vi "Check Default Plugins.vi"(8 "error in (no error)":errorcluster, 11 "Configuration Manager in":refnum<class "Configuration Manager.lvclass">) -> (0 "error out":errorcluster, 3 "Configuration Manager out":refnum<class "Configuration Manager.lvclass">)   [LabVIEW 2020, in "Configuration Manager.lvclass"]
uses:
  Configuration Manager.lvclass
  Configuration Manager.lvclass/Configuration Manager.ctl
  <vilib>/Utility/config.llb/NI_LVConfig.lvlib
  <vilib>/Utility/config.llb/Read Key (Boolean).vi
  <vilib>/Utility/config.llb/Write Key (Boolean).vi
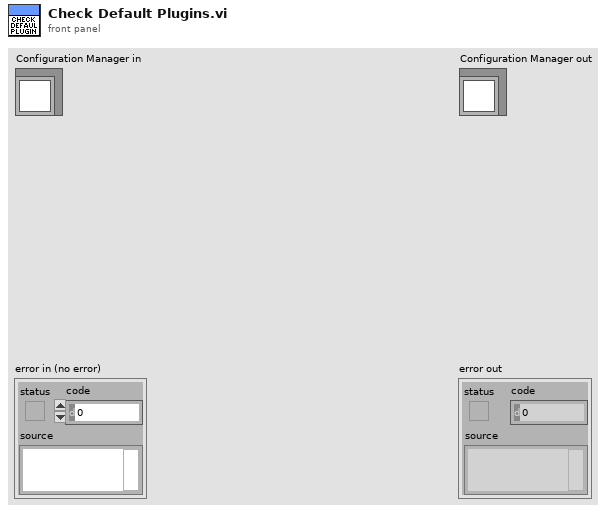
[diagram p1: front panel]
types:
  T1 = typedef "NI_LVConfig.lvlib/Config Data RefNum.ctl" = refnum<k1>
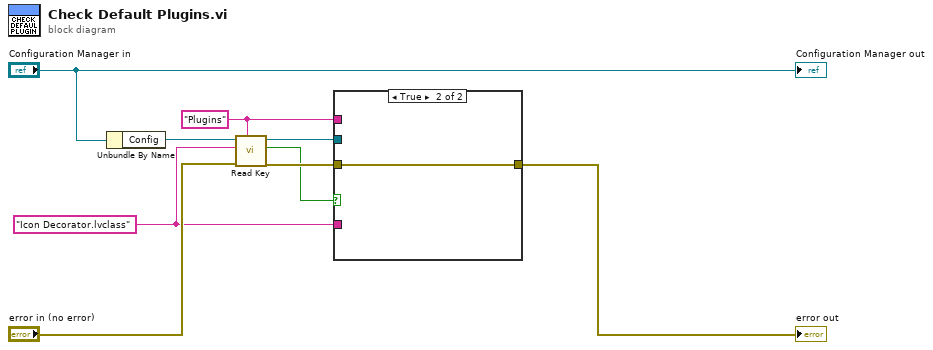
[diagram p0: block diagram]
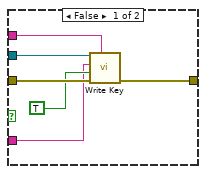
[diagram p2: hidden frame]
diagram:
  w2 = "Icon Decorator.lvclass" ("key")
  w1 = "Plugins" ("section")
  n1 = Unbundle By Name("Configuration Manager in") -> ("Config"=w9:T1)
  n2 = call-poly <vilib>:"Read Key.vi"("section"=w1, "error in (no error)"="error in (no error)", "key"=w2, "refnum"=w9) -> ("error out"=w6:errorcluster, "found?"=w3:bool, "refnum out"=w7:T1)  [unwired: 4 in, 1 out]
  n3 = case shown="True" w3 {
    tunnel: w7 -> [w15 _]
    tunnel: w6 -> [w14 w16]
    tunnel: [w13 w16] -> w4
    tunnel: w2 -> [w11 _]
    tunnel: w1 -> [w10 _]
    frame False {
      n4 = call-poly <vilib>:"Write Key.vi"("section"=w10, "error in (no error)"=w14, "value"=TRUE, "key"=w11, "refnum"=w15) -> ("error out"=w13:errorcluster)  [unwired: 4 in, 2 out]
    }
    frame True {
    }
  }
  "error out" <- w4
  "Configuration Manager out" <- "Configuration Manager in"
